vi "Cache SC2250 Session.vi"(0 "Instrument name":string, 5 "sc2250 session in":refnum<k15>, 11 "error in (no error)":errorcluster) -> (4 "sc2250 session out":refnum<k15>, 15 "error out":errorcluster)   [LabVIEW 2023, in "RFFixtureCharact.RFPM.lvlib" / "SG SC2250 Path Group.lvclass"]
uses:
  SG SC2250 Path Group.lvclass
  Common/Data Cache/Type Definitions/Dictionary Operation.ctl
  Common/RFCalAndFixtureCharact.Common.lvlib
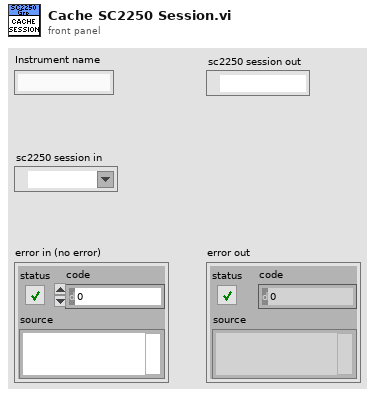
[diagram p1: front panel]
types:
  T1 = typedef "RFCalAndFixtureCharact.Common.lvlib/Dictionary Operation.ctl" = enum16{"Read", "Insert", "Remove", "Clear", "Get All", "Update"}
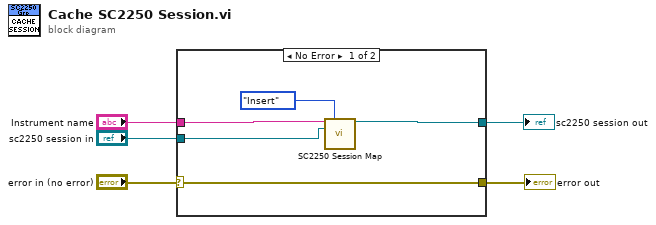
[diagram p0: block diagram]
diagram:
  n1 = case shown="No Error" "error in (no error)" {
    selector: "error in (no error)" -> [w10 w12]
    tunnel: [w10 w12] -> w4
    tunnel: "Instrument name" -> [w9 _]
    tunnel: "sc2250 session in" -> [w7 w11]
    tunnel: [w6 w11] -> w1
    frame No Error {
      n2 = call "SC2250 Session Map.vi"("Instrument name"=w9, "Action"=Dictionary_Operation."Insert", "sc2250 session in"=w7) -> ("sc2250 session"=w6:refnum<k15>)  [unwired: 10 in, 2 out]
    }
    frame Error {
    }
  }
  "error out" <- w4
  "sc2250 session out" <- w1
